vi "Process.vi"(8 "error in":errorcluster, 11 "Plugin in":refnum<class "Dynamic Channel.lvclass">) -> (0 "error out":errorcluster, 3 "Plugin out":refnum<class "Dynamic Channel.lvclass">)   [LabVIEW 2020, in "Dynamic Channel.lvlib" / "Dynamic Channel.lvclass"]
uses:
  Dynamic Channel.lvclass
  C:/Program Files/National Instruments/LabVIEW 2020/vi.lib/FlexLogger/SDK/PluginSDK.lvlibp/PEFClasses/SDK/Plugin/Plugin.lvclass
  <vilib>/FlexLogger/SDK/PluginSDK.lvlibp/PEFClasses/SDK/Producer Channel/Producer Channel.lvclass
  C:/Program Files/National Instruments/LabVIEW 2020/vi.lib/FlexLogger/SDK/PluginSDK.lvlibp/PEFClasses/SDK/Channel/Channel.lvclass
  <vilib>/FlexLogger/SDK/PluginSDK.lvlibp/PEFClasses/SDK/Plugin/Get Waveform.vi
  <vilib>/FlexLogger/SDK/PluginSDK.lvlibp/PEFClasses/SDK/Channel/ParameterAccess/Read DBL.vi
  <vilib>/FlexLogger/SDK/PluginSDK.lvlibp/PEFClasses/SDK/Plugin/DataHelpers/Write 1D Wfm (DBL).vi
  <vilib>/FlexLogger/SDK/PluginSDK.lvlibp/PEFClasses/SDK/Plugin/Plugin.lvclass
  <vilib>/FlexLogger/SDK/PluginSDK.lvlibp/PEFClasses/SDK/Channel/Channel.lvclass
  C:/Program Files/National Instruments/LabVIEW 2020/vi.lib/FlexLogger/SDK/PluginSDK.lvlibp/PEFClasses/SDK/Processing Element/Processing Element.lvclass
  C:/Users/Localization Tester/Documents/LabVIEW Projects/FlexLogger IO Plugins/Dynamic Channel/Dynamic Channel.lvclass
  C:/Program Files/National Instruments/LabVIEW 2020/vi.lib/FlexLogger/SDK/PluginSDK.lvlibp/PEFClasses/SDK/Producer Channel/Producer Channel.lvclass
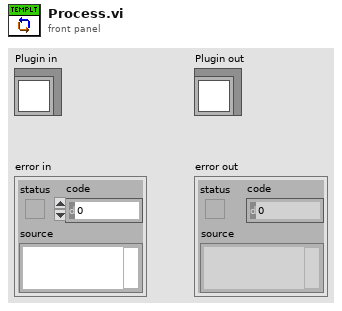
[diagram p1: front panel]
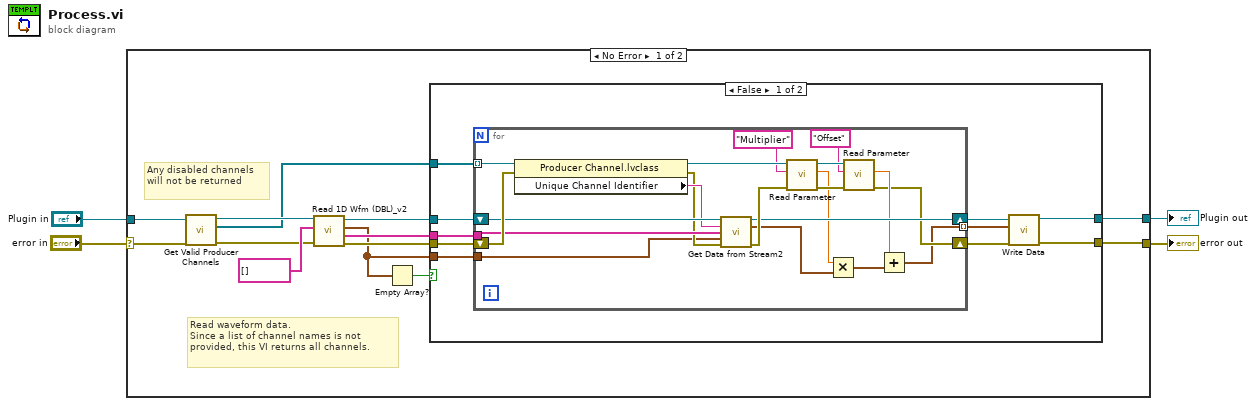
[diagram p0: block diagram]
diagram:
  n1 = case shown="No Error" "error in" {
    selector: "error in" -> [w15 w50]
    tunnel: [w6 w51] -> w1
    tunnel: "Plugin in" -> [w16 w51]
    tunnel: [w5 w50] -> w2
    frame No Error {
      # "Any disabled channels will not be returned"
      # "Read waveform data.\nSince a list of channel names is not provided, this VI returns all channels."
      n2 = call <vilib>:"Get Valid Producer Channels.vi"("error in (no error)"=w15, "Plugin in"=w16) -> ("error out"=w13:errorcluster, "Channels"=w8:refnum<class "Producer Channel.lvclass">[], "Plugin out"=w14:refnum<class "Dynamic Channel.lvclass">)  [unwired: 7 in]
      n3 = call <vilib>:"Read 1D Wfm (DBL)_v2.vi"("error in (no error)"=w13, "Unique Identifers (empty = all)"=string[] [] ("Unique Channel Identifers (empty = all)"), "Plugin in"=w14) -> ("error out"=w10:errorcluster, "Stream Names"=w9:string[], "Data"=w7:waveform(dbl)[], "Plugin out"=w11:refnum<class "Dynamic Channel.lvclass">)  [unwired: 5 in]
      n4 = Empty Array?(array=w7) -> (empty?=w12:bool)
      n5 = case shown="False" w12 {
        tunnel: w11 -> [w25 w49]
        tunnel: w10 -> [w26 w48]
        tunnel: w9 -> [w24 _]
        tunnel: w8 -> [w27 _]
        tunnel: w7 -> [w23 _]
        tunnel: [w19 w49] -> w6
        tunnel: [w18 w48] -> w5
        frame False {
          n6 = for {
            tunnel: w27 -> [w47] mode=indexing
            shift-right: [w29] -> w21
            shift-left: w26 -> [w46]
            shift-right: [w37] -> w22
            shift-left: w25 -> [w45]
            tunnel: w24 -> [w43]
            tunnel: w23 -> [w41]
            tunnel: [w28] -> w20 mode=indexing
            n7 = property class="Producer Channel.lvclass"(reference=w47, error in=w46) -> (reference out=w39:refnum<class "Producer Channel.lvclass">, error out=w42:errorcluster, "Unique Channel Identifier"=w44:string)
            n8 = call-poly <vilib>:"Get Data from Stream2.vi"("Plugin in"=w45, "Unique Identifier"=w44, "Stream Names"=w43, "Stream Values"=w41, "error in (no error)"=w42) -> ("Plugin out"=w37:refnum<class "Dynamic Channel.lvclass">, "Waveform"=w33:waveform(dbl), "error out"=w40:errorcluster)  [unwired: 7 in, 1 out]
            n9 = call-poly <vilib>:"Read Parameter.vi"("error in (no error)"=w40, "Name"="Multiplier", "Channel in"=w39) -> ("error out"=w36:errorcluster, "Value"=w32:dbl, "Channel out"=w35:refnum<class "Producer Channel.lvclass">)  [unwired: 5 in, 1 out]
            n10 = Multiply(x=w32, y=w33) -> (x*y=w31:waveform(dbl))
            n11 = call-poly <vilib>:"Read Parameter.vi"("error in (no error)"=w36, "Name"="Offset", "Channel in"=w35) -> ("error out"=w29:errorcluster, "Value"=w30:dbl)  [unwired: 5 in, 2 out]
            n12 = Add(x=w30, y=w31) -> (x+y=w28:waveform(dbl))
          }
          n13 = call-poly <vilib>:"Write Data.vi"("error in (no error)"=w21, "Data"=w20, "Plugin in"=w22) -> ("error out"=w18:errorcluster, "Plugin out"=w19:refnum<class "Dynamic Channel.lvclass">)  [unwired: 7 in]
        }
        frame True {
        }
      }
    }
    frame Error {
    }
  }
  "error out" <- w2
  "Plugin out" <- w1
